vi "setUnits.vi"(8 "error in (no error)":errorcluster, 10 "units":string, 11 "ACNET Device in":refnum<class "Copy of ACNET Device.lvclass">) -> (0 "error out":errorcluster, 3 "ACNET Device out":refnum<class "Copy of ACNET Device.lvclass">)   [LabVIEW 2013, in "Copy of ACNET Device.lvclass"]
uses:
  Copy of ACNET Device.lvclass
  Copy of ACNET Device.lvclass/Copy of ACNET Device.ctl
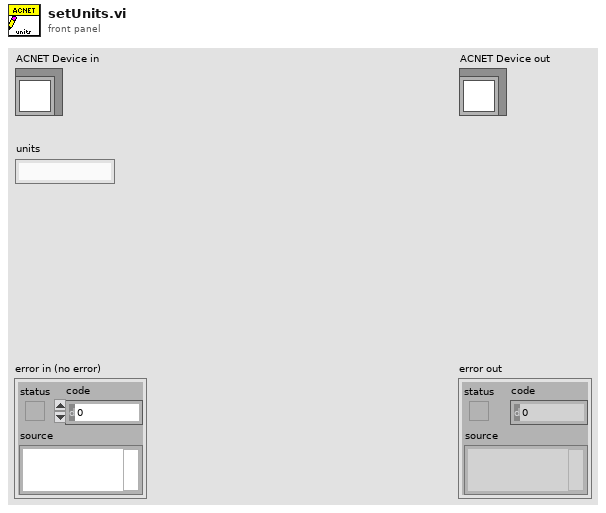
[diagram p1: front panel]
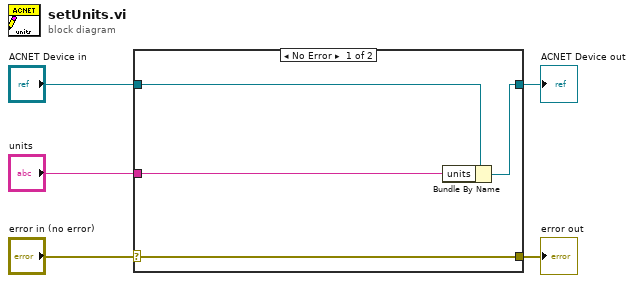
[diagram p0: block diagram]
diagram:
  n1 = case shown="No Error" "error in (no error)" {
    selector: "error in (no error)" -> [w9 w10]
    tunnel: [w9 w10] -> w4
    tunnel: [w7 w11] -> w2
    tunnel: "ACNET Device in" -> [w8 w11]
    tunnel: "units" -> [w6 _]
    frame No Error {
      n2 = Bundle By Name(cluster=w8, "units"=w6) -> (w7:refnum<class "Copy of ACNET Device.lvclass">)
    }
    frame Error {
    }
  }
  "error out" <- w4
  "ACNET Device out" <- w2
